vi "sub_loopcount.vi"(7 "cmd":enum16{"ini", "count 1", "read"}(ring)) -> (3 "countn":u32)   [LabVIEW 2018]
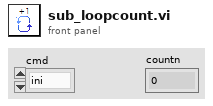
[diagram p1: front panel]
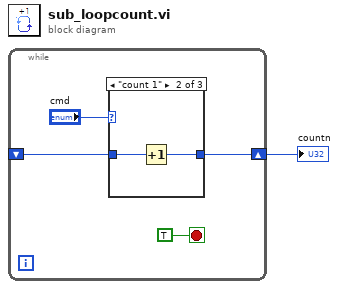
[diagram p0: block diagram]
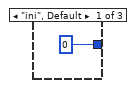
[diagram p2: hidden frame]
diagram:
  n1 = while {
    shift-right: [w3] -> w1
    shift-left: _ -> [w2]
    stop <- TRUE stop-if-true
    n2 = case shown="\"count 1\"" "cmd" {
      tunnel: [u32 0 w7 w9] -> w3
      tunnel: w2 -> [_ w8 w9]
      frame "ini", Default {
      }
      frame "count 1" {
        n3 = Increment(x=w8) -> (x+1=w7:u32)
      }
      frame "read" {
      }
    }
  }
  "countn" <- w1
